vi "CheckNames.vi"(6 "BD":T1 items=["Server", "Local DB"], 8 "error in":errorcluster, 9 "Value in":string, 10 "DB in":T2, 11 "Path":path) -> (0 "error out":errorcluster, 2 "DB out":T2, 3 "Value out":string)   [LabVIEW 2019]
uses:
  <vilib>/addons/database/Connection.llb/Conn ObjectReference.ctl
  TypeDef/#TypeDef_DBMode.ctl
  <vilib>/addons/database/NI_Database_API.lvlib
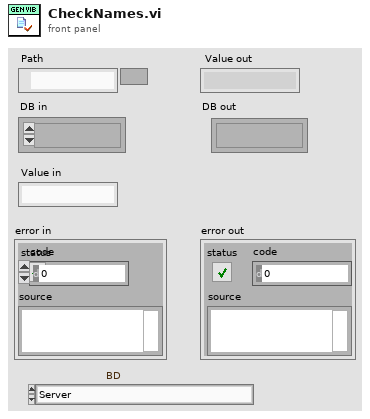
[diagram p1: front panel]
types:
  T1 = typedef "#TypeDef_DBMode.ctl" = u16
  T2 = typedef "NI_Database_API.lvlib/Conn ObjectReference.ctl" = refnum<k1>
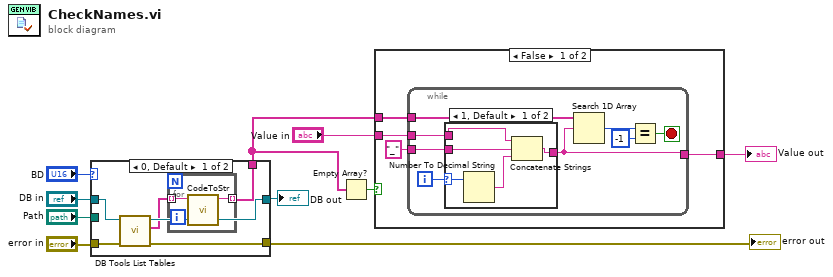
[diagram p0: block diagram]
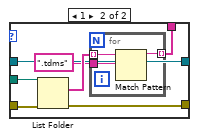
[diagram p2: hidden frame]
diagram:
  n1 = case shown="0, Default" "BD" {
    tunnel: [w13 w25] -> w10
    tunnel: [w11 w24] -> w5
    tunnel: "error in" -> [w14 w21]
    tunnel: "Path" -> [_ w20]
    tunnel: "DB in" -> [w16 w19]
    tunnel: [w15 w19] -> w1
    frame 0, Default {
      n2 = call <vilib>:"DB Tools List Tables.vi"("error in (no error)"=w14, "connection reference"=w16) -> ("error out"=w13:errorcluster, "tables"=w12:string[], "connection reference out"=w15:T2)  [unwired: 3 in]
      n3 = for {
        tunnel: w12 -> [w18] mode=indexing
        tunnel: [w17] -> w11 mode=indexing
        n4 = call "CodeToStr.vi"("Name in"=w18) -> ("Name out"=w17:string)  [unwired: 10 in]
      }
    }
    frame 1 {
      n5 = List Folder(path=w20, error in=w21) -> (filenames=w23:string[], error out=w25:errorcluster)  [unwired: 2 in, 2 out]
      n6 = for {
        tunnel: w23 -> [w28] mode=indexing
        tunnel: [w27] -> w24 mode=indexing
        tunnel: ".tdms" -> [w26]
        n7 = Match Pattern(string=w28, regular expression=w26) -> (before substring=w27:string)  [unwired: 1 in, 3 out]
      }
    }
  }
  "error out" <- w10
  "DB out" <- w1
  n8 = Empty Array?(array=w5) -> (empty?=w4:bool)
  n9 = case shown="False" w4 {
    tunnel: w5 -> [w32 _]
    tunnel: "Value in" -> [w31 w47]
    tunnel: [w29 w47] -> w8
    frame False {
      n10 = while {
        tunnel: w32 -> [w40]
        tunnel: w31 -> [w37]
        tunnel: "_" ("string") -> [w39]
        tunnel: [w36] -> w29
        i -> [w38]
        stop <- w33 stop-if-true
        n11 = case shown="1, Default" w38 {
          selector: w38 -> [w44 _]
          tunnel: w39 -> [w45 _]
          tunnel: w37 -> [w42 w46]
          tunnel: [w41 w46] -> w36
          frame 1, Default {
            n12 = Number To Decimal String(number=w44) -> (decimal integer string=w43:string)  [unwired: 1 in]
            n13 = Concatenate Strings(w42, w45, w43) -> (w41:string)
          }
          frame 0 {
          }
        }
        n14 = Search 1D Array(1D array=w40, element=w36) -> (index of element=w35:i32)  [unwired: 1 in]
        n15 = Equal?(x=w35, y=-1) -> (x = y?=w33:bool)
      }
    }
    frame True {
    }
  }
  "Value out" <- w8
